vi "generate_voltage_lists.vi"(0 "MinVoltage":dbl=1.0, 1 "Initial sweep direction":u16(ring) items=["Low to high", "High to low"], 5 "Max Voltage":dbl=2.0, 7 "Measurement Delay (ms)":dbl=100.0, 9 "V step":dbl, 11 "t step":dbl, 12 "NPLC":dbl) -> (6 "Voltage Forward List":dbl[](array[numeric]), 8 "Settling delay (s)":dbl, 10 "Voltage Reverse List":dbl[](array[numeric]))   [LabVIEW 2016]
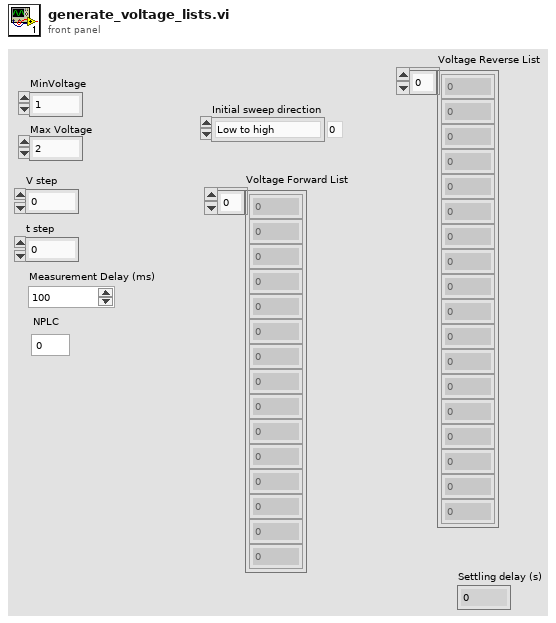
[diagram p1: front panel]
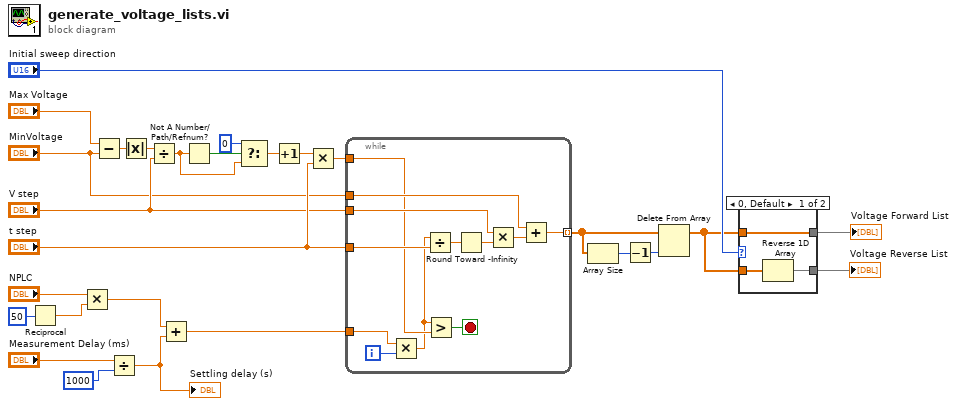
[diagram p0: block diagram]
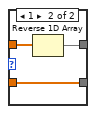
[diagram p2: hidden frame]
diagram:
  n1 = Reciprocal(x=50) -> (1/x=w18:dbl)
  n2 = Multiply(x="NPLC", y=w18) -> (x*y=w9:dbl)
  n3 = Subtract(x="Max Voltage", y="MinVoltage") -> (x-y=w20:dbl)
  n4 = Divide(x="Measurement Delay (ms)", y=1000) -> (x/y=w6:dbl)
  "Settling delay (s)" <- w6
  n5 = Absolute Value(x=w20) -> (abs(x)=w21:dbl)
  n6 = Divide(x=w21, y="V step") -> (x/y=w25:dbl)
  n7 = Add(x=w9, y=w6) -> (x+y=w5:dbl)
  n8 = Not A Number/Path/Refnum?(number/path/refnum=w25) -> (NaN/Path/Refnum?=w27:bool)
  n9 = Select(t=0, s=w27, f=w25) -> (s? t:f=w24:dbl)
  n10 = Increment(x=w24) -> (x+1=w23:dbl)
  n11 = Multiply(x=w23, y="t step") -> (x*y=w13:dbl)
  n12 = while {
    tunnel: w5 -> [w39]
    tunnel: "t step" -> [w37]
    tunnel: "V step" -> [w34]
    tunnel: "MinVoltage" -> [w32]
    tunnel: w13 -> [w30]
    tunnel: [w28] -> w4 mode=indexing
    i -> [w38]
    stop <- w31 stop-if-true
    n13 = Multiply(x=w39, y=w38) -> (x*y=w29:dbl)
    n14 = Divide(x=w29, y=w37) -> (x/y=w36:dbl)
    n15 = Greater?(x=w29, y=w30) -> (0:w31:bool)
    n16 = Round Toward -Infinity(1:w36) -> (0:w35:dbl)
    n17 = Multiply(x=w34, y=w35) -> (x*y=w33:dbl)
    n18 = Add(x=w32, y=w33) -> (x+y=w28:dbl)
  }
  n19 = Array Size(array=w4) -> (size(s)=w2:i32)
  n20 = Decrement(x=w2) -> (x-1=w1:i32)
  n21 = Delete From Array(array=w4, index=w1) -> (array with subset deleted=w3:dbl[])  [unwired: 1 in, 1 out]
  n22 = case shown="0, Default" "Initial sweep direction" {
    tunnel: w3 -> [w41 w43]
    tunnel: [w40 w43] -> w10
    tunnel: [w42 w44] -> w11
    tunnel: w3 -> [w42 w45]
    frame 0, Default {
      n23 = Reverse 1D Array(array=w41) -> (reversed array=w40:dbl[])
    }
    frame 1 {
      n24 = Reverse 1D Array(array=w45) -> (reversed array=w44:dbl[])
    }
  }
  "Voltage Forward List" <- w11
  "Voltage Reverse List" <- w10
